vi "Write Current_Share.vi"(8 "error in":errorcluster, 10 "Current_Sharing":bool, 11 "PowerSupply in":refnum<class "PowerSupply.lvclass">) -> (0 "error out":errorcluster, 3 "PowerSupply out":refnum<class "PowerSupply.lvclass">)   [LabVIEW 2019, in "PowerSupply.lvlib" / "PowerSupply.lvclass"]
uses:
  Library/PowerSupply.lvclass
  C:/Users/Public/Documents/Development/builds/Instruments/Instruments.lvlibp/Library/Instruments.lvclass
  Library/PowerSupply.lvclass/PowerSupply.ctl
  Read Settings.vi
  Write Settings.vi
  builds/Instruments/Instruments.lvlibp/Private/Polymorphic/Special/Event from Boolean.vi
  builds/Instruments/Instruments.lvlibp/Accessors/Command with Logging.vi
  builds/Engine/Engine.lvlibp/Project/Engine.lvclass
  builds/Instruments/Instruments.lvlibp/Library/Instruments.lvclass
  builds/Instruments/Instruments.lvlibp
  C:/Users/Public/Documents/Development/builds/Engine/Engine.lvlibp/Project/Engine.lvclass
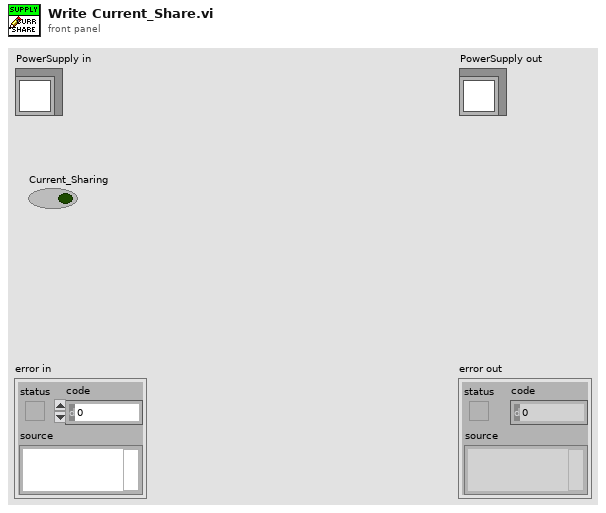
[diagram p1: front panel]
types:
  T1 = typedef "PowerSupply.lvlib/PowerSupply.lvclass/Settings.ctl" = cluster{"Voltage":dbl, "Current":dbl, "Output":bool, "OverVolt_Protect":dbl, "OverCurrent_Protect":dbl, "OVP":bool, "OCP":bool, "Interlock":bool, "Volt_Ramp":dbl, "Current_Ramp":dbl, "Sense Point":T2, "OCP Mode":T3, "Sharing":bool}
  T2 = typedef "PowerSupply.lvlib/PowerSupply.lvclass/Sense Point.ctl" = enum16{"Local", "Remote"}
  T3 = typedef "PowerSupply.lvlib/PowerSupply.lvclass/OCP Mode.ctl" = enum16{"Shutdown", "Foldback"}
  T4 = cluster{"Timestamp":timestamp, "Description":string, "Data":string}
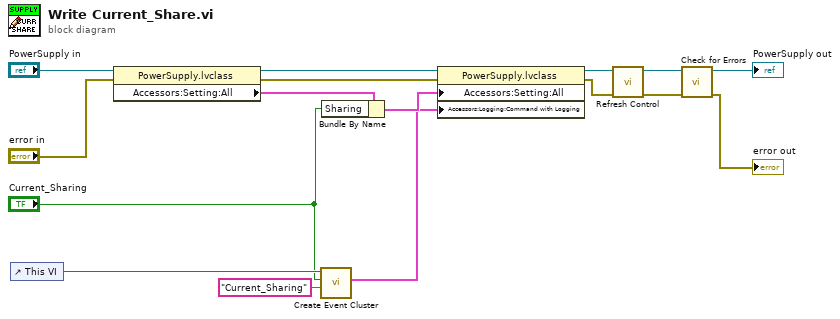
[diagram p0: block diagram]
diagram:
  n1 = control-ref of="This VI"() -> (w4:refnum<vi>)
  n2 = property class="PowerSupply.lvclass"(reference="PowerSupply in", error in="error in") -> (reference out=w16:refnum<class "PowerSupply.lvclass">, error out=w8:errorcluster, "Accessors:Setting:All"=w10:T1)
  n3 = call-poly "Create Event Cluster.vi"("Name"="Current_Sharing", "Value"="Current_Sharing", "VI Refnum"=w4) -> ("Event Data"=w1:T4)  [unwired: 8 in]
  n4 = Bundle By Name(cluster=w10, "Sharing"="Current_Sharing") -> (w9:T1)
  n5 = property class="PowerSupply.lvclass"(reference=w16, error in=w8, "Accessors:Setting:All"=w9, "Accessors:Logging:Command with Logging"=w1) -> (reference out=w15:refnum<class "PowerSupply.lvclass">, error out=w7:errorcluster)
  n6 = call "Refresh Control.vi"("error in"=w7, "PowerSupply in"=w15) -> ("error out"=w5:errorcluster, "PowerSupply out"=w6:refnum<class "PowerSupply.lvclass">)  [unwired: 8 in]
  n7 = call "Check for Errors.vi"("error in"=w5, "Engine in"=w6) -> ("error out"=→"error out":errorcluster, "Engine out"=→"PowerSupply out":refnum<class "PowerSupply.lvclass">)  [unwired: 8 in]
